vi "HM_times_x_preload.vi"(5 "SLMAX":fxp<+/-,18,5>, 6 "preload_addr":u8, 7 "primary_write_addr":u8, 8 "preload_vec":T1=[0.0, 0.0, 0.0, 0.0, 0.0, 0.0, 0.0, 0.0, 0.0, 0.0, 0.0, 0.0], 9 "Ns+StartIndex":u16, 10 "StartIndex":u8, 11 "x_vec":T3=[0.0, 0.0, 0.0, 0.0, 0.0, 0.0, 0.0, 0.0, 0.0, 0.0, 0.0, 0.0, 0.0, 0.0, 0.0, 0.0, 0.0, 0.0, 0.0, 0.0, 0.0, 0.0, 0.0, 0.0, 0.0]) -> (0 "done":bool, 2 "A*x":T1)   [LabVIEW 2017]
uses:
  x_vec_type_pipe.ctl
  x_qp_scalar.ctl
  ziyi_pipe.ctl
  <vilib>/Platform/TimedLoop/XDataNode/timing_clust.ctl
  <vilib>/Platform/TimedLoop/XDataNode/nitl_modes.ctl
  <vilib>/Platform/TimedLoop/XDataNode/wakeup.ctl
  <vilib>/rvi/Emulation/niFpgaSctlEmulationGetInTimedLoop.vi
  <vilib>/rvi/Emulation/niFpgaEmulationReportErrorSimple.vi
  <vilib>/rvi/Emulation/niFpgaGetClockAttributes.vi
  <vilib>/rvi/Emulation/niFpgaCriticalErrorInLSC.vi
  <vilib>/Platform/TimedLoop/XDataNode/XDataNode.xnode
  <vilib>/Platform/TimedLoop/XDataNode/XDNodeRunTimeDep.lvlib
panel:
  in  "Ns":i16
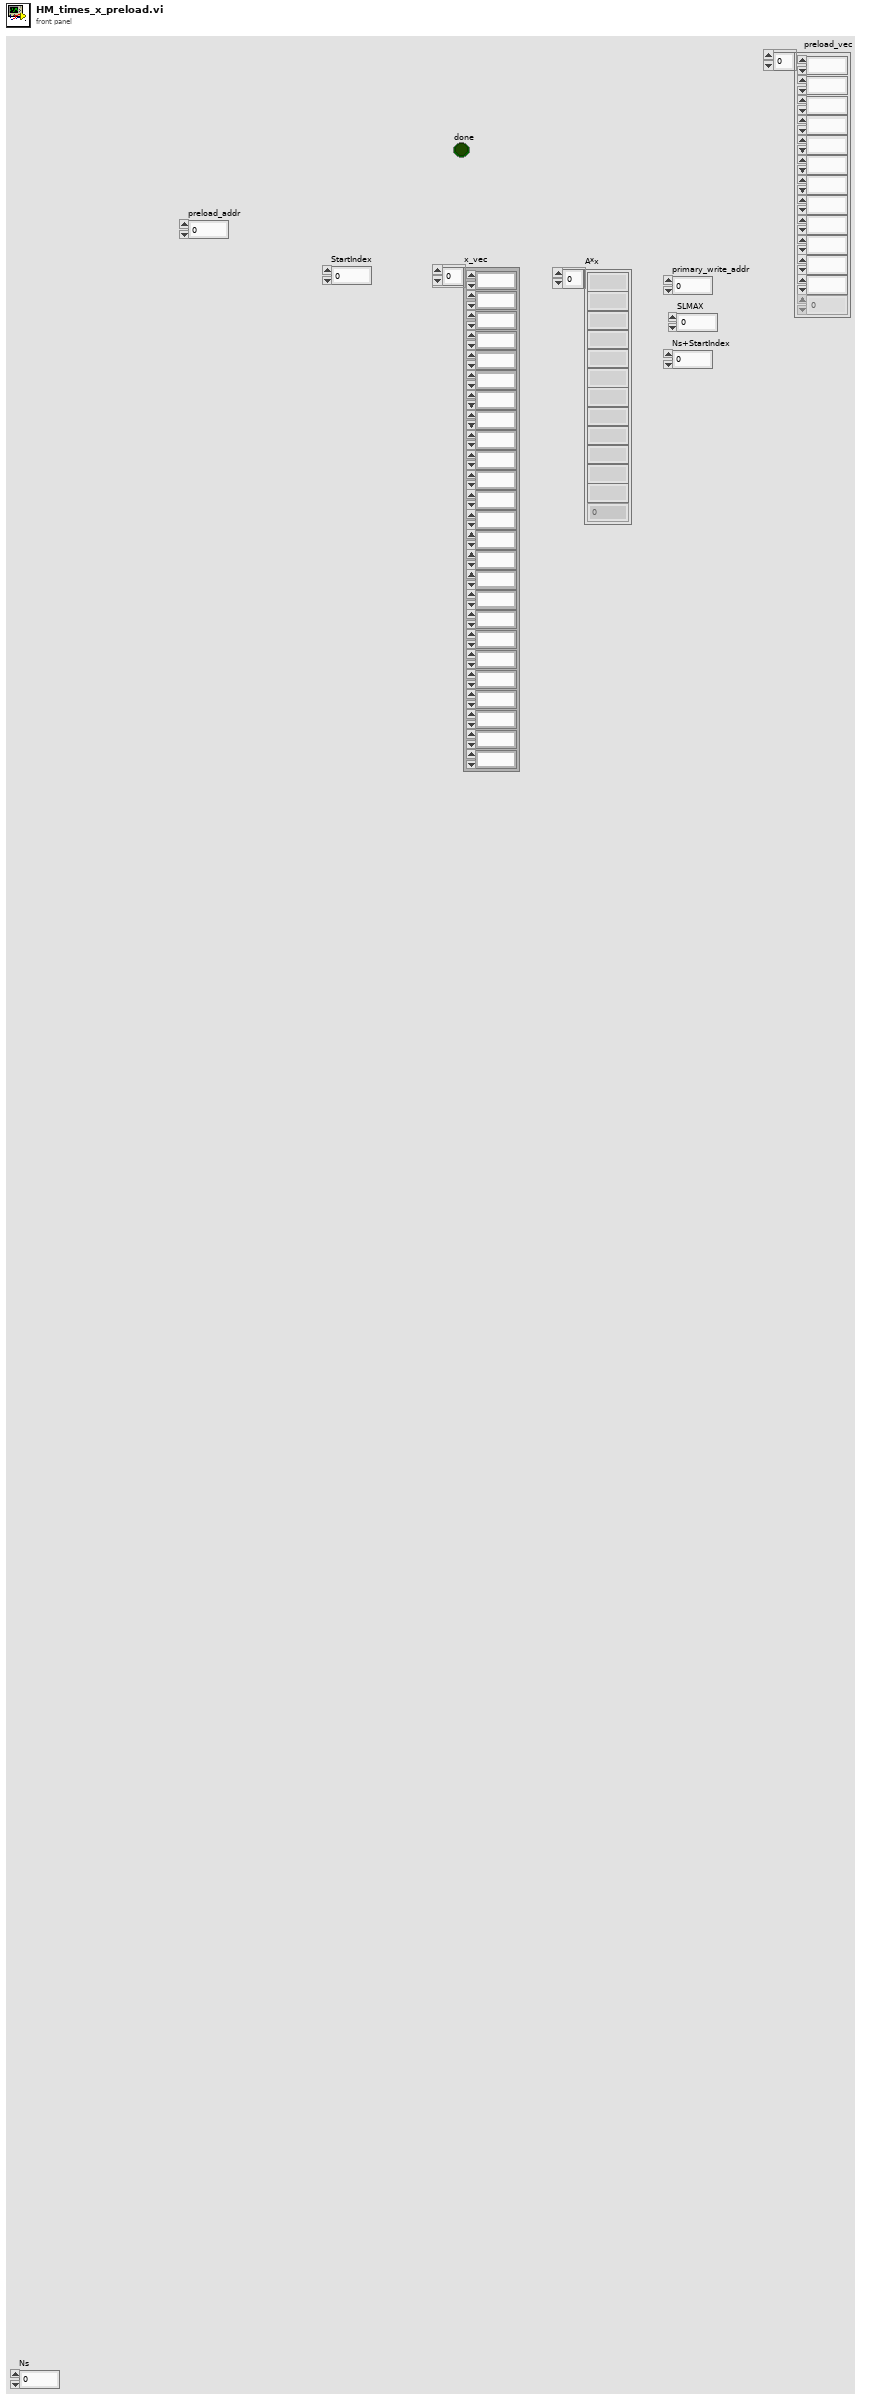
[diagram p1: front panel]
types:
  T1 = typedef "ziyi_pipe.ctl" = T2[]
  T2 = typedef "x_qp_scalar.ctl" = fxp<+/-,32,6>
  T3 = typedef "x_vec_type_pipe.ctl" = T2[]
  T4 = typedef "XDNodeRunTimeDep.lvlib/timing_clust.ctl" = cluster{"Expected End [f-1]":u64, "Actual End [f-1]":u64, "Finished Late? [f-1]":bool, "Expected End [i-1]":u64, "Actual End [i-1]":u64, "Finished Late? [i-1]":bool, "Expected Start [i]":u64, "Actual Start [i]":u64, "Expected Start [f]":u64, "Actual Start [f]":u64, "Source Name":string, "Structure Name":string, "Period":i64, "Deadline":i64, "Offset":i64, "Start":i64, "Priority":i32, "Timeout":i32, "Mode":T5, "Wakeup Reason":T6, "Error":errorcluster, "Source Type":string, "Secondary Source Type":string, "Global End Time":u64, "Global Start Time":u64, "Frame Duration":u64, "Iteration Duration":u64, "Assigned CPU":i32, "I/O Scan Engine Mode":u32}
  T5 = typedef "XDNodeRunTimeDep.lvlib/nitl_modes.ctl" = enum32{"No Change", "Process missed periods, maintain original phase", "Discard missed periods, maintain original phase", "Process missed periods, ignore original phase", "Discard missed periods, ignore original phase"}
  T6 = typedef "XDNodeRunTimeDep.lvlib/wakeup.ctl" = enum32{"Normal", "Aborted", "Asynchronous wakeup", "Timing source error", "Timed loop error", "Timeout"}
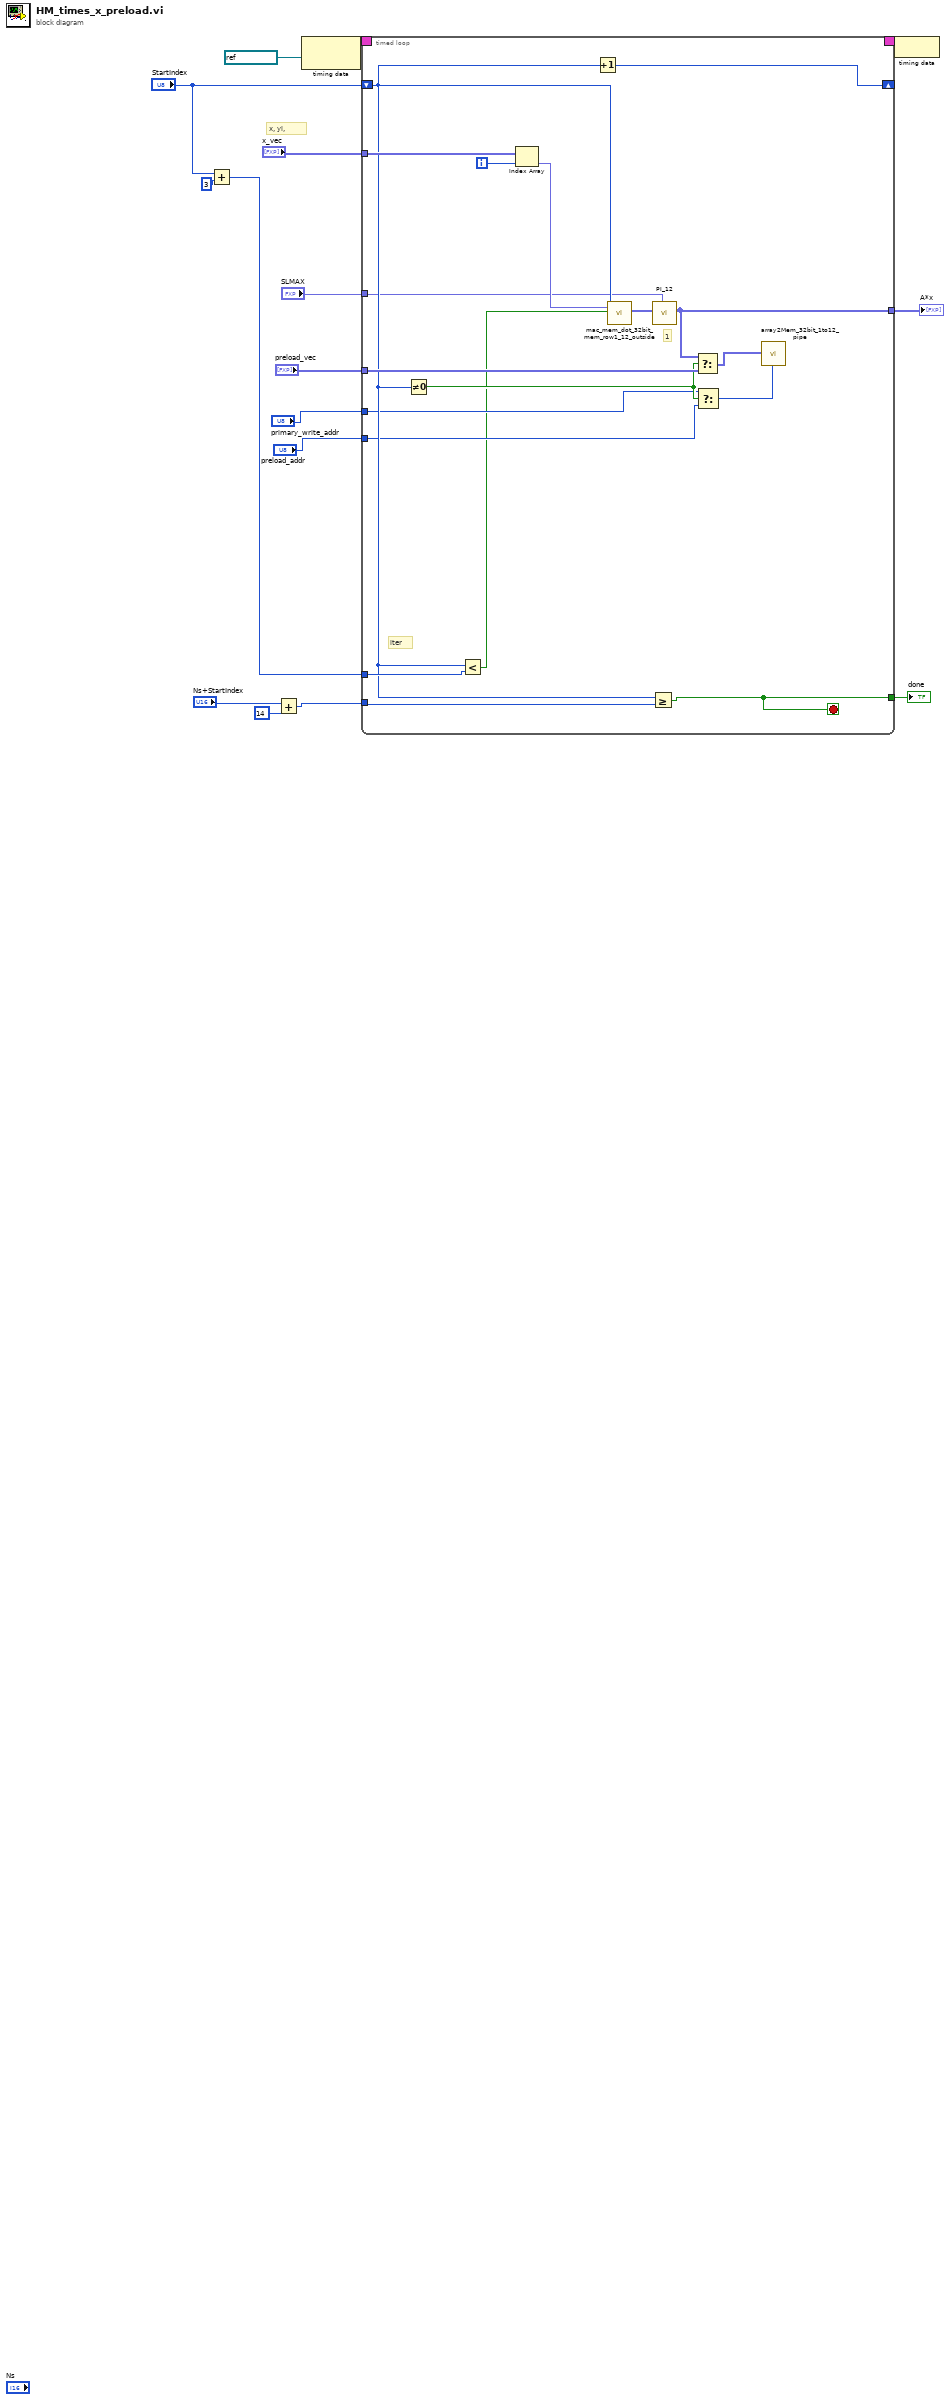
[diagram p0: block diagram]
diagram:
  # "x, yi,"
  n1 = Add(x="StartIndex", y=i16 3) -> (x+y=w11:i16)
  n2 = Add(x="Ns+StartIndex", y=u16 14) -> (x+y=w6:u16)
  n3 = node-c288(refnum<k21> "100MHz" ("Source Name")) -> (w16:T4)
  n4 = timed-loop {
    timing: w16 -> [_]
    timing-out: [_] -> w15
    tunnel: w6 -> [w34]
    shift-right: [w33] -> _
    shift-left: "StartIndex" -> [w26]
    tunnel: w11 -> [w31]
    tunnel: [w24] -> w2
    tunnel: "preload_vec" -> [w28]
    tunnel: "x_vec" -> [w32]
    tunnel: [w23] -> w10
    tunnel: "SLMAX" -> [w22]
    tunnel: "preload_addr" -> [w21]
    tunnel: "primary_write_addr" -> [w20]
    i -> [w18]
    stop <- w23 stop-if-true
    # "iter"
    # "1"
    n5 = Not Equal To 0?(x=w26) -> (x != 0?=w25:bool)
    n6 = Less?(x=w26, y=w31) -> (x < y?=w19:bool)
    n7 = Index Array(array=w32, index=w18) -> (element=w27:T2)
    n8 = Increment(x=w26) -> (x+1=w33:u8)
    n9 = call "mac_mem_dot_32bit_mem_row1_12_outside.vi"("StartIndex"=w26, "x_i"=w27, "Boolean"=w19) -> ("ziyi_type"=w17:T1)  [unwired: 16 in]
    n10 = Greater Or Equal?(x=w26, y=w34) -> (x >= y?=w23:bool)
    n11 = call "PI_12.vi"("SLMAX"=w22, "ziyi_f_in"=w17) -> ("ziyi_f_out"=w24:T1)  [unwired: 9 in]
    n12 = Select(t=w24, s=w25, f=w28) -> (s? t:f=w30:T1)
    n13 = Select(t=w20, s=w25, f=w21) -> (s? t:f=w29:u8)
    n14 = call "array2Mem_32bit_1to12_pipe.vi"("Address (Max = 255)"=w29, "array_in"=w30) -> ()  [unwired: 10 in]
  }
  "done" <- w10
  "A*x" <- w2
  n15 = node-c288(w15) -> ()
